vi "file_save.vi"(0 "Array":dbl[](array[numeric])) -> ()   [LabVIEW 2015]
panel:
  out "spreadsheet string":string
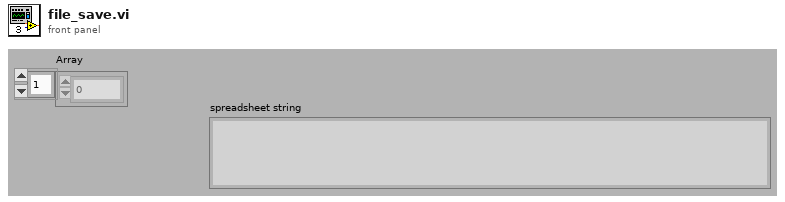
[diagram p1: front panel]
types:
  T1 = enum16{"open", "open or create", "create or replace", "create", "open (read only)"}
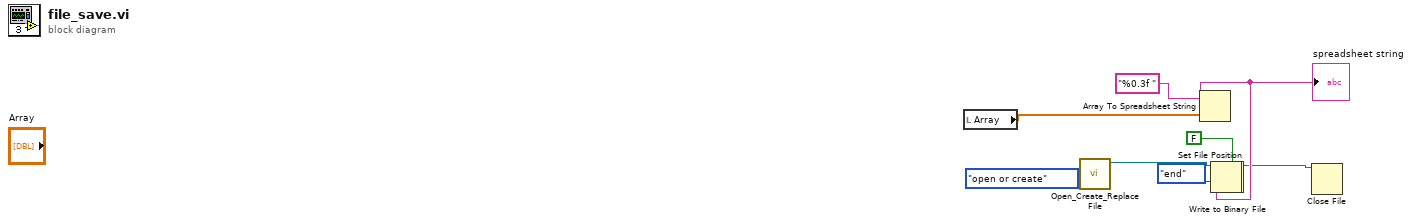
[diagram p0: block diagram]
diagram:
  n1 = local read "Array"() -> (w4:dbl[])
  n2 = call <vilib>:"Open_Create_Replace File.vi"("function (open:0)"=T1."open or create") -> ("refnum"=w8:refnum<file>)  [unwired: 7 in, 3 out]
  n3 = Array To Spreadsheet String(array=w4, 3:"%0.3f " ("format string")) -> (spreadsheet string=w6:string)  [unwired: 1 in]
  "spreadsheet string" <- w6
  n4 = Set File Position(refnum=w8, from (0:start)=enum16{"start", "end", "current"}."end" ("pos mode (0:2)")) -> (refnum out=w3:refnum<file>, error out=w2:errorcluster)  [unwired: 2 in]
  n5 = Write to Binary File(file (use dialog)=w3, data=w6, error in=w2, 5:FALSE ("预置数组或字符串大小？(T)")) -> (refnum out=w5:refnum<file>)  [unwired: 2 in, 2 out]
  n6 = Close File(refnum=w5) -> ()  [unwired: 1 in, 2 out]
